vi "CMN_GetFromDBS.vi"(10 "str in":string) -> (2 "str out":string)   [LabVIEW 2016]
uses:
  DBSHAND/private/vis/DatabaseHand_Element_Get(string).vi
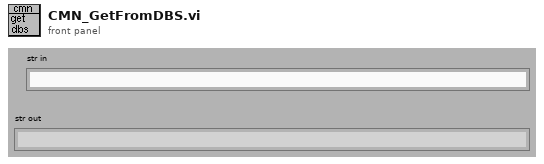
[diagram p1: front panel]
types:
  T1 = typedef "DatabaseHand_RefNum.ctl" = refnum<vi>
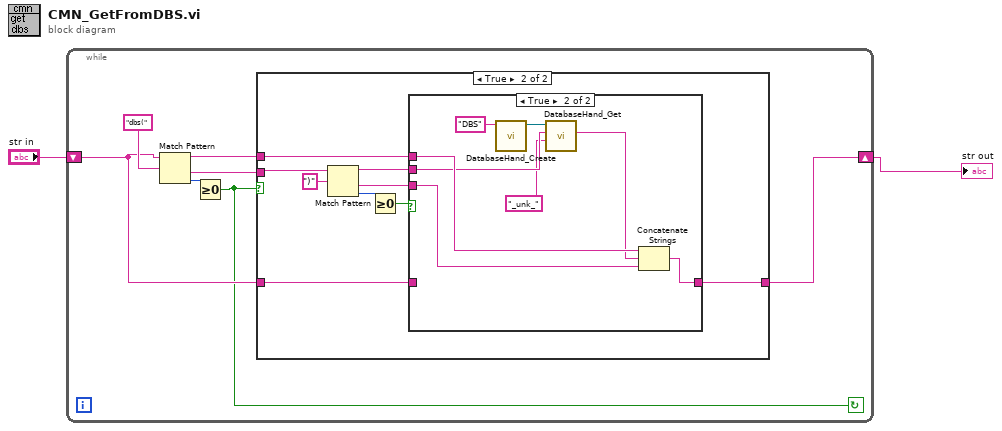
[diagram p0: block diagram]
diagram:
  n1 = while {
    shift-right: [w4] -> w1
    shift-left: "str in" -> [w5]
    stop <- w3 continue-if-true
    n2 = Match Pattern(string=w5, regular expression="dbs(" ("x")) -> (before substring=w6:string, after substring=w7:string, offset past match=w9:i32)  [unwired: 2 out]
    n3 = Greater Or Equal To 0?(x=w9) -> (x >= 0?=w3:bool)
    n4 = case shown="True" w3 {
      tunnel: w5 -> [w10 w15]
      tunnel: [w10 w14] -> w4
      tunnel: w7 -> [_ w19]
      tunnel: w6 -> [_ w12]
      frame False {
      }
      frame True {
        n5 = Match Pattern(string=w19, regular expression=")") -> (before substring=w13:string, after substring=w11:string, offset past match=w17:i32)  [unwired: 2 out]
        n6 = Greater Or Equal To 0?(x=w17) -> (x >= 0?=w16:bool)
        n7 = case shown="True" w16 {
          tunnel: w15 -> [w20 _]
          tunnel: [w20 w27] -> w14
          tunnel: w13 -> [_ w22]
          tunnel: w12 -> [_ w28]
          tunnel: w11 -> [_ w24]
          frame False {
          }
          frame True {
            n8 = call "DatabaseHand_Create.vi"("Name"="DBS") -> ("Database RefNum out"=w25:T1)  [unwired: 1 in, 9 out]
            n9 = call-poly "DatabaseHand_Get.vi"("default value"="_unk_", "name"=w22, "Database RefNum in"=w25) -> ("value"=w23:string)  [unwired: 2 in, 6 out]
            n10 = Concatenate Strings(w28, w23, w24) -> (w27:string)
          }
        }
      }
    }
  }
  "str out" <- w1
